vi "Get DataRow (String).vi"(8 "error in (no error)":errorcluster, 10 "index":i32, 11 "DataGridView in":refnum<class "DataGridView.lvclass">) -> (0 "error out":errorcluster, 2 "Array":string[](array[string]), 3 "DataGridView out":refnum<class "DataGridView.lvclass">)   [LabVIEW 2016, in "DataGrid.lvlib" / "DataGridView.lvclass"]
uses:
  <userlib>/LabVIEWdotNetDataGrid/source/DataGridView/DataGridView.lvclass
  <userlib>/LabVIEWdotNetDataGrid/source/DataGridView/DataGridView.lvclass/DataGridView.ctl
  <userlib>/LabVIEWdotNetDataGrid/source/DataTable/DataTable.lvclass
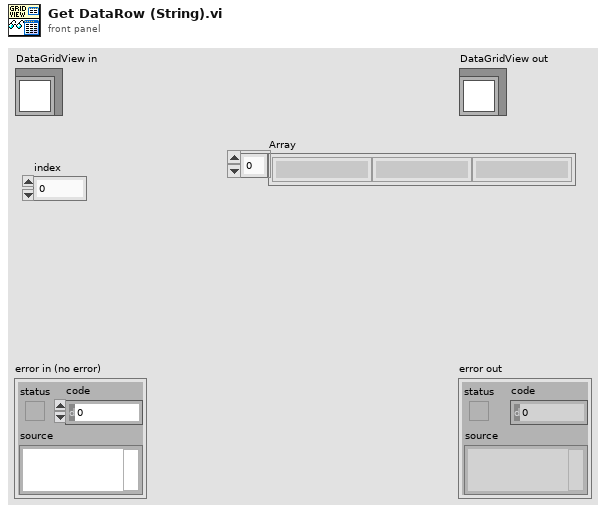
[diagram p1: front panel]
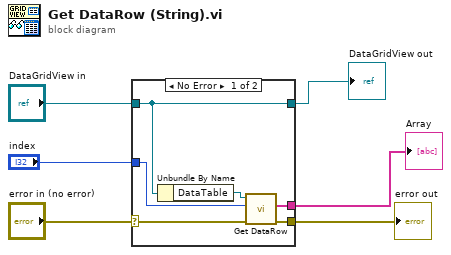
[diagram p0: block diagram]
diagram:
  n1 = case shown="No Error" "error in (no error)" {
    selector: "error in (no error)" -> [w10 w13]
    tunnel: [w9 w13] -> w5
    tunnel: [w12 w14] -> w3
    tunnel: "DataGridView in" -> [w12 w14]
    tunnel: [w8 _] -> w2
    tunnel: "index" -> [w7 _]
    frame No Error {
      n2 = Unbundle By Name(w12) -> ("DataTable"=w11:refnum<class "DataTable.lvclass">)
      n3 = call-poly <userlib>:"Get DataRow.vi"("error in (no error)"=w10, "index"=w7, "DataTable in"=w11) -> ("error out"=w9:errorcluster, "Array"=w8:string[])  [unwired: 6 in, 1 out]
    }
    frame Error {
    }
  }
  "error out" <- w5
  "DataGridView out" <- w3
  "Array" <- w2
